vi "myTask.vi"(8 "error in (no error)":errorcluster, 10 "stopMechanism":refnum<class "ITaskChannel.lvclass">, 11 "ITask in":refnum<class "ITask.lvclass">) -> (0 "error out":errorcluster, 3 "ITask out":refnum<class "ITask.lvclass">)   [LabVIEW 2023, in "Task_BoolStopNotifier.lvclass"]
uses:
  Task_BoolStopNotifier.lvclass
  ITask/ITask.lvclass
  ITaskChannel/ITaskChannel.lvclass
  C:/projects/TLC_Daemon/source/ITask/ITask.lvclass
  Task_BoolStopNotifier.lvclass/Task_BoolStopNotifier.ctl
  BoolNotifierTaskChannel/BoolNotifierTaskChannel.lvclass/BoolNotifierTaskChannel.ctl
  Write loopCounter.vi
  NotifierStopMechanism/Read notifierRef.vi
  Read description.vi
  TLC_Daemon.lvlib
  C:/projects/TLC_Daemon/source/Examples/Example_Bool_Notifier_StopMech/Task_BoolStopNotifier/Task_BoolStopNotifier.lvclass
panel:
  out "loopCounter":i32 caption="Loop Counter"
  out "description":string
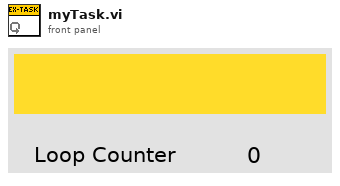
[diagram p1: front panel]
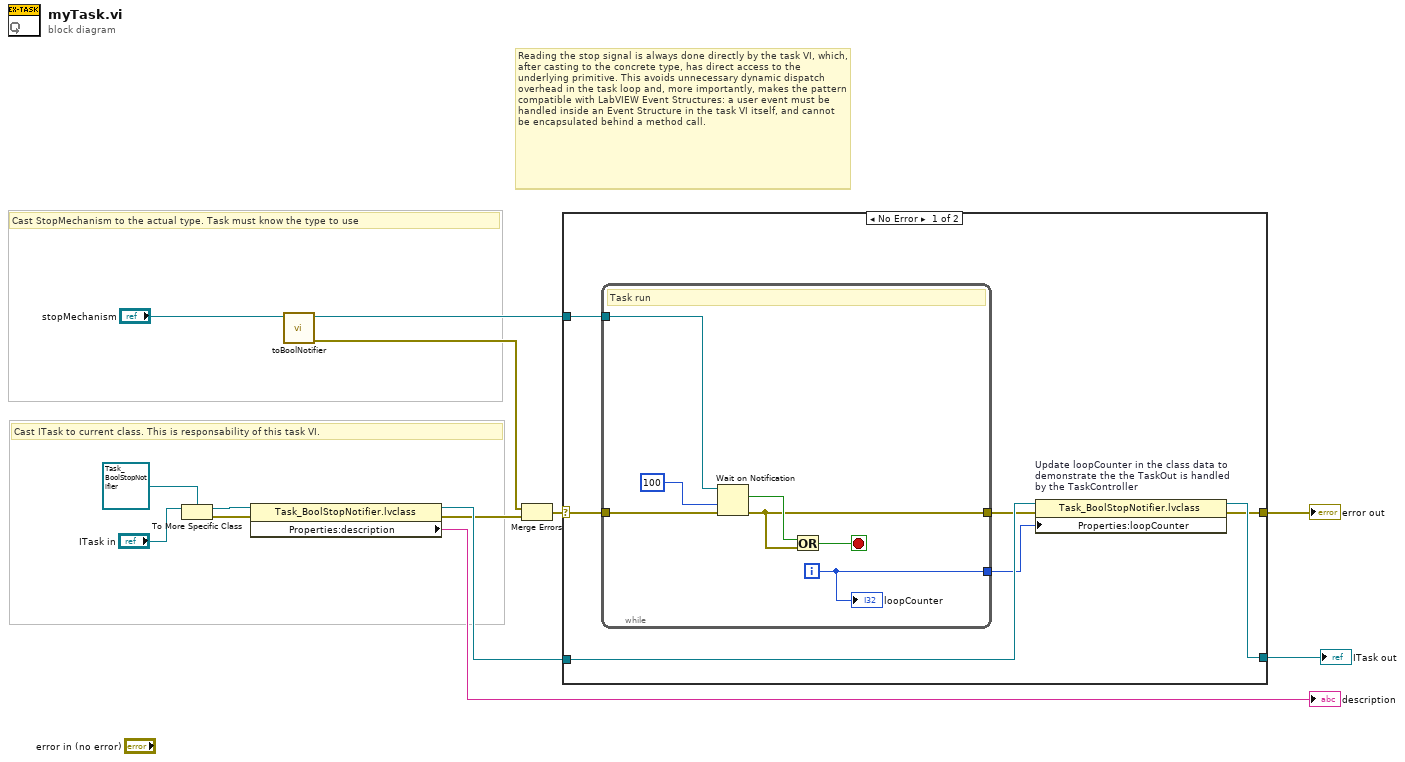
[diagram p0: block diagram]
diagram:
  # "Reading the stop signal is always done directly by the task VI, which, after casting to the concrete type, has direct access to the underlying primitive. This avoids unnecessary dynamic dispatch overhead in the task loop and, more importantly, makes the pattern compatible with LabVIEW Event Structures: a user event must be handled inside an Event Structure in the task VI itself, and cannot be encapsulated behind a method call."
  # "Reading the stop signal is always done directly by the task VI, which, after casting to the concrete type, has direct access to the underlying primitive. This avoids unnecessary dynamic dispatch overhead in the task loop and, more importantly, makes the pattern compatible with LabVIEW Event Structures: a user event must be handled inside an Event Structure in the task VI itself, and cannot be encapsulated behind a method call."
  # "Cast ITask to current class. This is responsability of this task VI."
  # "Cast StopMechanism to the actual type. Task must know the type to use"
  n1 = To More Specific Class(target class=refnum<class "Task_BoolStopNotifier.lvclass"> refnum ("ExampleTask_StopNotifier.lvclass"), reference="ITask in") -> (specific class reference=w9:refnum<class "Task_BoolStopNotifier.lvclass">, error out=w10:errorcluster)  [unwired: 1 in]
  n2 = property class="Task_BoolStopNotifier.lvclass"(reference=w9, error in=w10) -> (reference out=w6:refnum<class "Task_BoolStopNotifier.lvclass">, error out=w4:errorcluster, "Properties:description"=→"description":string)
  n3 = call "toBoolNotifier.vi"("ITaskChannel"="stopMechanism") -> ("error out"=w3:errorcluster, "boolNotifier"=w7:refnum<notifier>)  [unwired: 9 in]
  n4 = Merge Errors(w3, w4) -> (w2:errorcluster)
  n5 = case shown="No Error" w2 {
    selector: w2 -> [w16 w29]
    tunnel: w7 -> [w20 _]
    tunnel: w6 -> [w19 w28]
    tunnel: [w17 w28] -> w5
    tunnel: [w14 w29] -> w1
    frame No Error {
      n6 = while {
        tunnel: w20 -> [w27]
        tunnel: w16 -> [w23]
        tunnel: [w22] -> w15
        tunnel: [w21] -> w18
        i -> [w21]
        stop <- w24 stop-if-true
        # "Task run"
        n7 = Wait on Notification(notifier=w27, timeout in ms (-1)=100, error in (no error)=w23) -> (notification=w25:bool, error out=w22:errorcluster)  [unwired: 1 in, 2 out]
        n8 = Or(x=w25, y=w22) -> (x .or. y?=w24:bool)
        "loopCounter" <- w21
      }
      n9 = property on="Update loopCounter in the class data to\ndemonstrate the the TaskOut is handled\nby the TaskController" class="Task_BoolStopNotifier.lvclass"(reference=w19, error in=w15, "Properties:loopCounter"=w18) -> (reference out=w17:refnum<class "Task_BoolStopNotifier.lvclass">, error out=w14:errorcluster)
    }
    frame Error {
    }
  }
  "error out" <- w1
  "ITask out" <- w5
